vi "Init.vi"(3 "Container State":T5, 4 "Previous State":variant=variant(cluster{"Current Channels Info":cluster{"Channel Name":string, "Used?":bool, "Alias":string, "Property Bundle":cluster{"Name":string, "Value":variant}[]}[], "Previous Channels Info":cluster{"Channel Name":string, "Used?":bool, "Alias":string, "Property Bundle":cluster{"Name":string, "Value":variant}[]}[], "Help Prefix":string, "Max Display Size":i32, "Max Size":i32, "Hide Buttons":bool} {"Current Channels Info"=[{"Channel Name"="A/AI0", "Used?"=TRUE, "Alias"="", "Property Bundle"=[{"Name"="Pin Annotation", "Value"=variant(string[] ["(Pin 3)", "", "", ""])}]}, {"Channel Name"="A/AI1", "Used?"=FALSE, "Alias"="", "Property Bundle"=[{"Name"="Pin Annotation", "Value"=variant(string[] ["(Pin 5)", "", "", ""])}]}, {"Channel Name"="A/AI2", "Used?"=FALSE, "Alias"="", "Property Bundle"=[{"Name"="Pin Annotation", "Value"=variant(string[] ["(Pin 7)", "", "", ""])}]}, {"Channel Name"="A/AI3", "Used?"=FALSE, "Alias"="", "Property Bundle"=[{"Name"="Pin Annotation", "Value"=variant(string[] ["(Pin 9)", "", "", ""])}]}, {"Channel Name"="B/AI0", "Used?"=FALSE, "Alias"="", "Property Bundle"=[{"Name"="Pin Annotation", "Value"=variant(string[] ["(Pin 3)", "", "", ""])}]}, {"Channel Name"="B/AI1", "Used?"=FALSE, "Alias"="", "Property Bundle"=[{"Name"="Pin Annotation", "Value"=variant(string[] ["(Pin 5)", "", "", ""])}]}, {"Channel Name"="B/AI2", "Used?"=FALSE, "Alias"="", "Property Bundle"=[{"Name"="Pin Annotation", "Value"=variant(string[] ["(Pin 7)", "", "", ""])}]}, {"Channel Name"="B/AI3", "Used?"=FALSE, "Alias"="", "Property Bundle"=[{"Name"="Pin Annotation", "Value"=variant(string[] ["(Pin 9)", "", "", ""])}]}, {"Channel Name"="C/AI0", "Used?"=FALSE, "Alias"="", "Property Bundle"=[{"Name"="Pin Annotation", "Value"=variant(string[] ["(AI0)", "", "", ""])}]}, {"Channel Name"="C/AI1", "Used?"=FALSE, "Alias"="", "Property Bundle"=[{"Name"="Pin Annotation", "Value"=variant(string[] ["(AI1)", "", "", ""])}]}, {"Channel Name"="AudioIn/Left", "Used?"=FALSE, "Alias"="", "Property Bundle"=[{"Name"="Pin Annotation", "Value"=variant(string[] ["", "", "", ""])}]}, {"Channel Name"="AudioIn/Right", "Used?"=FALSE, "Alias"="", "Property Bundle"=[{"Name"="Pin Annotation", "Value"=variant(string[] ["", "", "", ""])}]}], "Previous Channels Info"=[{"Channel Name"="A/AI0", "Used?"=FALSE, "Alias"="", "Property Bundle"=[{"Name"="Pin Annotation", "Value"=variant(string[] ["(Pin 3)", "", "", ""])}]}, {"Channel Name"="A/AI1", "Used?"=FALSE, "Alias"="", "Property Bundle"=[{"Name"="Pin Annotation", "Value"=variant(string[] ["(Pin 5)", "", "", ""])}]}, {"Channel Name"="A/AI2", "Used?"=FALSE, "Alias"="", "Property Bundle"=[{"Name"="Pin Annotation", "Value"=variant(string[] ["(Pin 7)", "", "", ""])}]}, {"Channel Name"="A/AI3", "Used?"=FALSE, "Alias"="", "Property Bundle"=[{"Name"="Pin Annotation", "Value"=variant(string[] ["(Pin 9)", "", "", ""])}]}, {"Channel Name"="B/AI0", "Used?"=FALSE, "Alias"="", "Property Bundle"=[{"Name"="Pin Annotation", "Value"=variant(string[] ["(Pin 3)", "", "", ""])}]}, {"Channel Name"="B/AI1", "Used?"=FALSE, "Alias"="", "Property Bundle"=[{"Name"="Pin Annotation", "Value"=variant(string[] ["(Pin 5)", "", "", ""])}]}, {"Channel Name"="B/AI2", "Used?"=FALSE, "Alias"="", "Property Bundle"=[{"Name"="Pin Annotation", "Value"=variant(string[] ["(Pin 7)", "", "", ""])}]}, {"Channel Name"="B/AI3", "Used?"=FALSE, "Alias"="", "Property Bundle"=[{"Name"="Pin Annotation", "Value"=variant(string[] ["(Pin 9)", "", "", ""])}]}, {"Channel Name"="C/AI0", "Used?"=FALSE, "Alias"="", "Property Bundle"=[{"Name"="Pin Annotation", "Value"=variant(string[] ["(AI0)", "", "", ""])}]}, {"Channel Name"="C/AI1", "Used?"=FALSE, "Alias"="", "Property Bundle"=[{"Name"="Pin Annotation", "Value"=variant(string[] ["(AI1)", "", "", ""])}]}, {"Channel Name"="AudioIn/Left", "Used?"=FALSE, "Alias"="", "Property Bundle"=[{"Name"="Pin Annotation", "Value"=variant(string[] ["", "", "", ""])}]}, {"Channel Name"="AudioIn/Right", "Used?"=FALSE, "Alias"="", "Property Bundle"=[{"Name"="Pin Annotation", "Value"=variant(string[] ["", "", "", ""])}]}], "Help Prefix"="AI", "Max Display Size"=10, "Max Size"=12, "Hide Buttons"=FALSE}), 5 "Previous Version":T4={"Major"=1, "Minor"=0, "Fix"=0, "Build"=0}) -> (2 "Current State":T1={"Current Channels Info"=[{"Channel Name"="A/AI0", "Alias"="", "Used?"=FALSE, "Not Support?"=FALSE, "Property Bundle"=[]}, {"Channel Name"="A/AI1", "Alias"="", "Used?"=FALSE, "Not Support?"=FALSE, "Property Bundle"=[]}, {"Channel Name"="A/AI2", "Alias"="", "Used?"=FALSE, "Not Support?"=FALSE, "Property Bundle"=[]}, {"Channel Name"="A/AI3", "Alias"="", "Used?"=FALSE, "Not Support?"=FALSE, "Property Bundle"=[]}, {"Channel Name"="B/AI0", "Alias"="", "Used?"=FALSE, "Not Support?"=FALSE, "Property Bundle"=[]}, {"Channel Name"="B/AI1", "Alias"="", "Used?"=FALSE, "Not Support?"=FALSE, "Property Bundle"=[]}, {"Channel Name"="B/AI2", "Alias"="", "Used?"=FALSE, "Not Support?"=FALSE, "Property Bundle"=[]}, {"Channel Name"="B/AI3", "Alias"="", "Used?"=FALSE, "Not Support?"=FALSE, "Property Bundle"=[]}, {"Channel Name"="C/AI0", "Alias"="", "Used?"=FALSE, "Not Support?"=FALSE, "Property Bundle"=[]}, {"Channel Name"="C/AI1", "Alias"="", "Used?"=FALSE, "Not Support?"=FALSE, "Property Bundle"=[]}, {"Channel Name"="AudioIn/Left", "Alias"="", "Used?"=FALSE, "Not Support?"=FALSE, "Property Bundle"=[]}, {"Channel Name"="AudioIn/Right", "Alias"="", "Used?"=FALSE, "Not Support?"=FALSE, "Property Bundle"=[]}], "Help Prefix"="", "Max Display Size"=8, "Max Size"=10, "Show Buttons"=TRUE, "Data Valid"=refnum, "Show Range"=FALSE, "Range Items"=[], "Range Index"=[]})   [LabVIEW 2021, in "myRIO Channel List.xctl"]
uses:
  <vilib>/myRIO/Common/Express VI Framework/xctls/myRIO Channel List/myRIO Channel List.xctl
  <vilib>/myRIO/Common/Express VI Framework/xctls/myRIO Channel List/State.ctl
  <vilib>/myRIO/Common/Profile Manager Framework/typedefs/Channel Info.ctl
  <vilib>/myRIO/Common/Express VI Framework/typedefs/Data Validate Ref.ctl
  <vilib>/_xctls/Container State.ctl
  <vilib>/_xctls/Version.ctl
  <vilib>/_xctls/XControlSupport.lvlib
panel:
  in  "Default Indicator State":T1={"Current Channels Info"=[], "Help Prefix"="", "Max Display Size"=8, "Max Size"=0, "Show Buttons"=TRUE, "Data Valid"=refnum, "Show Range"=FALSE, "Range Items"=[], "Range Index"=[]}
  in  "Default Control State":T1={"Current Channels Info"=[], "Help Prefix"="", "Max Display Size"=8, "Max Size"=0, "Show Buttons"=TRUE, "Data Valid"=refnum, "Show Range"=FALSE, "Range Items"=[], "Range Index"=[]}
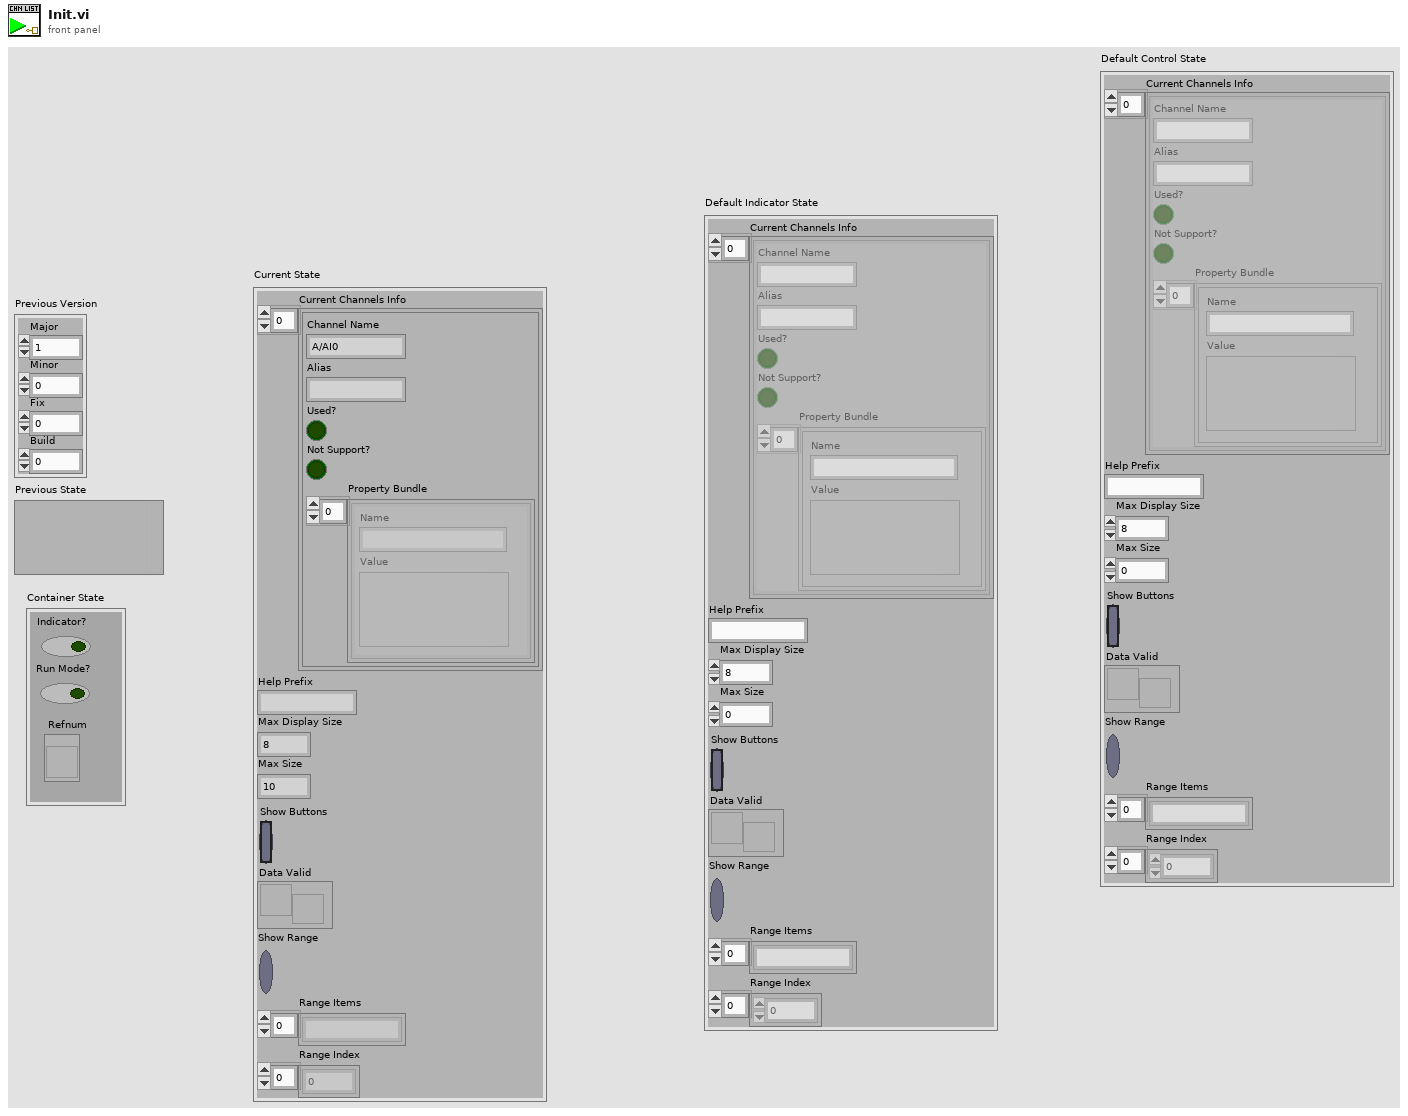
[diagram p1: front panel]
types:
  T1 = typedef "myRIO Channel List.xctl/State.ctl" = cluster{"Current Channels Info":T2[], "Help Prefix":string, "Max Display Size":i32, "Max Size":i32, "Show Buttons":bool, "Data Valid":T3, "Show Range":bool, "Range Items":string[], "Range Index":i32[]}
  T2 = typedef "Channel Info.ctl" = cluster{"Channel Name":string, "Alias":string, "Used?":bool, "Not Support?":bool, "Property Bundle":cluster{"Name":string, "Value":variant}[]}
  T3 = typedef "Data Validate Ref.ctl" = refnum<user-event>
  T4 = typedef "XControlSupport.lvlib/Version.ctl" = cluster{"Major":u16, "Minor":u16, "Fix":u16, "Build":u16}
  T5 = typedef "XControlSupport.lvlib/Container State.ctl" = cluster{"Indicator?":bool, "Run Mode?":bool, " Refnum":refnum<vi>}
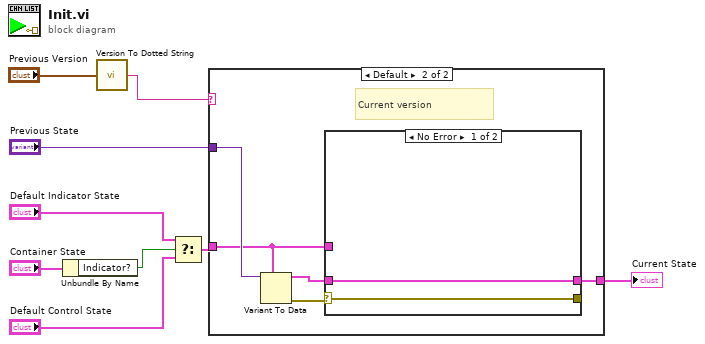
[diagram p0: block diagram]
diagram:
  n1 = Unbundle By Name("Container State") -> ("Indicator?"=w4:bool)
  n2 = call <vilib>:"Version To Dotted String.vi"("Version"="Previous Version") -> ("String Version"=w1:string)
  n3 = Select(t="Default Indicator State", s=w4, f="Default Control State") -> (s? t:f=w3:T1)
  n4 = case shown="Default" w1 {
    tunnel: "Previous State" -> [_ w15]
    tunnel: [w10 w11] -> w8
    tunnel: w3 -> [w10 w12]
    frame "0.0.0.0" {
      # "Just created, use default state"
    }
    frame Default {
      # "Current version"
      n5 = Variant To Data(type=w12, Variant=w15) -> (data=w13:T1, error out=w14:errorcluster)  [unwired: 1 in]
      n6 = case shown="No Error" w14 {
        selector: w14 -> [w17 w18]
        tunnel: w13 -> [w16 _]
        tunnel: [w16 w19] -> w11
        tunnel: w12 -> [_ w19]
        tunnel: [w17 w18] -> _
        frame No Error {
        }
        frame Error {
          # "Error converting previously \nsaved state. Use default instead."
        }
      }
    }
  }
  "Current State" <- w8
